vi "IPC-Modbus-Transfer-EncodeResponse-WriteMulRegisters.vi"(10 "Quantity of registers":u16, 11 "Starting Address":u16) -> (3 "输出字符串":string)   [LabVIEW 2014]
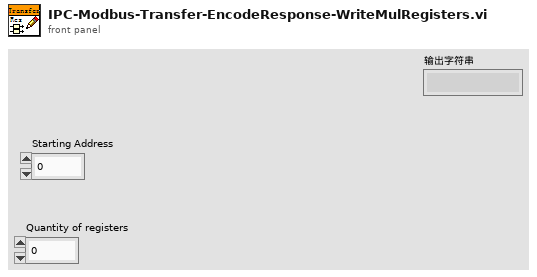
[diagram p1: front panel]
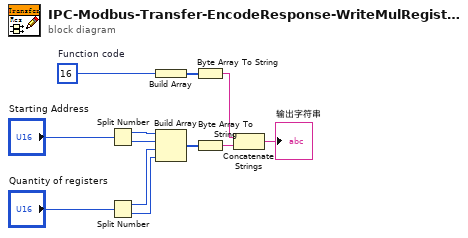
[diagram p0: block diagram]
diagram:
  w11 = u8 16  # Function code
  n1 = Split Number(x="Starting Address") -> (hi(x)=w5:u8, lo(x)=w4:u8)
  n2 = Split Number(x="Quantity of registers") -> (hi(x)=w3:u8, lo(x)=w2:u8)
  n3 = Build Array(w11) -> (w12:u8[])
  n4 = Build Array(w5, w4, w3, w2) -> (w1:u8[])
  n5 = Byte Array To String(unsigned byte array=w12) -> (string=w10:string)
  n6 = Byte Array To String(unsigned byte array=w1) -> (string=w9:string)
  n7 = Concatenate Strings(w10, w9) -> (→"输出字符串":string)
